vi "Write Data.vi"(8 "error in (no error)":errorcluster caption="entrée d'erreur (pas d'erreur)", 11 "Database Altyor en entrée":refnum<class "Database Altyor Packaging.lvclass">) -> (0 "error out":errorcluster caption="sortie d'erreur", 3 "Database Altyor en sortie":refnum<class "Database Altyor Packaging.lvclass">)   [LabVIEW 2020, in "Library Instrument & Equipement.lvlib" / "Library Database.lvlib" / "Database Altyor Packaging.lvclass"]
uses:
  Database Altyor Packaging.lvclass
  C:/Users/ngarcin/OneDrive - Altyor/Standard TB/Suite TB45/Class/Database/Database drivers/Database Drivers.lvclass
  Commun VI/TypeDef/Variable Printable.ctl
  Commun VI/Library Commun.lvlib
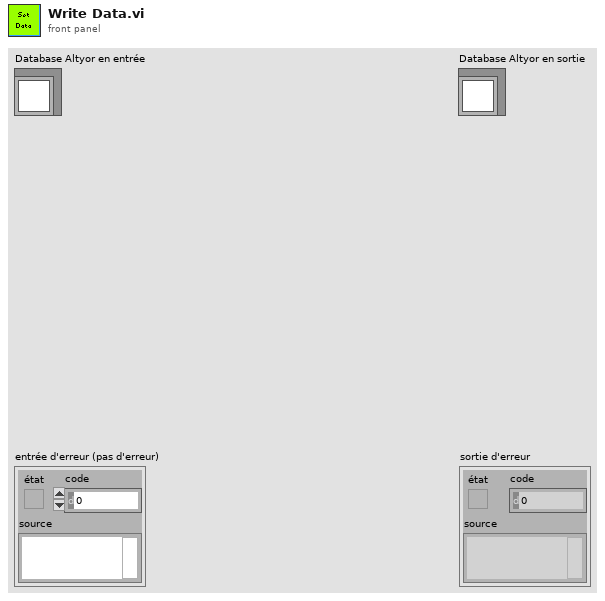
[diagram p1: front panel]
types:
  T1 = typedef "Variable Printable.ctl" = string
  T2 = enum16{"Get Variable", "Get All Variables", "Set Variable", "Delete Variable", "Delete All Variable"}
  T3 = cluster{"idPackaging":u32, "CreationDate":string, "EndOfProduction":string, "OrderNumber":string, "Batch":string, "PartNumber":string, "SerialNumber":string, "Operator":string, "Provisionning":string, "AdditionalInformation":string}
  T4 = cluster{"idPackaging":u32, "CreationDate":string, "EndOfProduction":string, "OrderNumber":string, "Batch":string, "PartNumber":string, "SerialNumber":string, "Operator":string, "Provisionning":string, "AdditionalInformation":string}[]
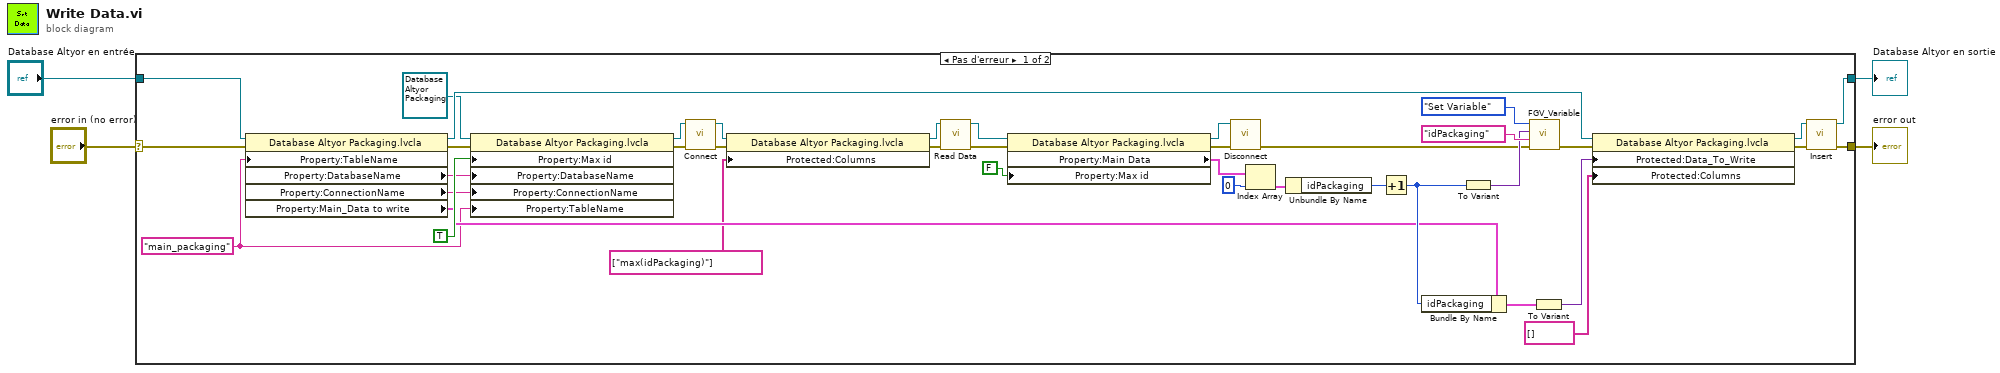
[diagram p0: block diagram]
diagram:
  n1 = case shown="Pas d'erreur" "error in (no error)" {
    selector: "error in (no error)" -> [w38 w45]
    tunnel: [w40 w45] -> w3
    tunnel: [w41 w44] -> w1
    tunnel: "Database Altyor en entrée" -> [w39 w44]
    frame No Error {
      w10 = "main_packaging" ("TableName")
      n2 = property class="Database Altyor Packaging.lvcla"(reference=w39, error in=w38, "Property:TableName"=w10) -> (reference out=w19:refnum<class "Database Altyor Packaging.lvclass">, error out=w14:errorcluster, "Property:DatabaseName"=w20:string, "Property:ConnectionName"=w21:string, "Property:Main_Data to write"=w11:T3)
      n3 = property class="Database Altyor Packaging.lvcla"(reference=refnum<class "Database Altyor Packaging.lvclass"> refnum ("Library Database.lvlib:Database Altyor.lvclass"), error in=w14, "Property:Max id"=TRUE ("Max id"), "Property:DatabaseName"=w20, "Property:ConnectionName"=w21, "Property:TableName"=w10) -> (reference out=w12:refnum<class "Database Altyor Packaging.lvclass">, error out=w13:errorcluster)
      n4 = call-dynamic "Connect.vi"("error in (no error)"=w13, "Database Altyor en entrée"=w12) -> ("error out"=w7:errorcluster, "Database Altyor en sortie"=w8:refnum<class "Database Altyor Packaging.lvclass">)  [unwired: 8 in]
      n5 = property class="Database Altyor Packaging.lvcla"(reference=w8, error in=w7, "Protected:Columns"=string[] ["max(idPackaging)"]) -> (reference out=w5:refnum<class "Database Altyor Packaging.lvclass">, error out=w6:errorcluster)
      n6 = call-dynamic "Read Data.vi"("error in (no error)"=w6, "Database Altyor en entrée"=w5) -> ("error out"=w31:errorcluster, "Database Altyor en sortie"=w32:refnum<class "Database Altyor Packaging.lvclass">)  [unwired: 8 in]
      n7 = property class="Database Altyor Packaging.lvcla"(reference=w32, error in=w31, "Property:Max id"=FALSE ("Max id")) -> (reference out=w18:refnum<class "Database Altyor Packaging.lvclass">, error out=w17:errorcluster, "Property:Main Data"=w30:T4)
      n8 = call-dynamic "Disconnect.vi"("error in (no error)"=w17, "Database Altyor en entrée"=w18) -> ("error out"=w16:errorcluster)  [unwired: 8 in, 1 out]
      n9 = Index Array(array=w30, index=0 ("indice")) -> (element=w36:T3)
      n10 = Unbundle By Name(w36) -> ("idPackaging"=w34:u32)
      n11 = Increment(x=w34) -> (x+1=w27:u32)
      n12 = Bundle By Name(cluster=w11, "idPackaging"=w27) -> (w33:T3)
      n13 = To Variant(anything=w27) -> (Variant=w26:variant)
      n14 = call "FGV_Variable.vi"("error in (no error)"=w16, "Variable"=T1 "idPackaging", "Data In"=w26, "Function"=T2."Set Variable") -> ("error out"=w25:errorcluster)  [unwired: 5 in, 2 out]
      n15 = To Variant(anything=w33) -> (Variant=w37:variant)
      n16 = property class="Database Altyor Packaging.lvcla"(reference=w19, error in=w25, "Protected:Data_To_Write"=w37, "Protected:Columns"=string[] [] ("Columns")) -> (reference out=w43:refnum<class "Database Altyor Packaging.lvclass">, error out=w42:errorcluster)
      n17 = call-dynamic "Insert.vi"("error in (no error)"=w42, "Database Drivers en entrée"=w43) -> ("error out"=w40:errorcluster, "Database Drivers en sortie"=w41:refnum<class "Database Altyor Packaging.lvclass">)  [unwired: 8 in]
    }
    frame Error {
    }
  }
  "error out" <- w3
  "Database Altyor en sortie" <- w1
